vi "Get Request Type.vi"(8 "error in (no error)":errorcluster, 11 "SetProfileParameter in":refnum<class "SetProfileParameter.lvclass">) -> (0 "error out":errorcluster, 2 "Request Type":string, 3 "SetProfileParameter out":refnum<class "SetProfileParameter.lvclass">)   [LabVIEW 2022 SP3, in "obs-websocket-lv.lvlib" / "SetProfileParameter.lvclass"]
uses:
  SetProfileParameter.lvclass
  SetProfileParameter.lvclass/SetProfileParameter.ctl
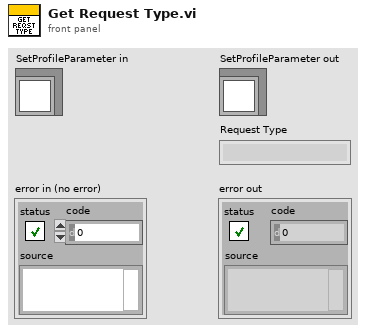
[diagram p1: front panel]
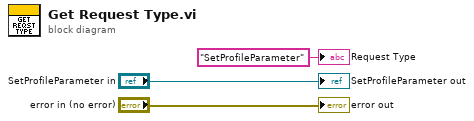
[diagram p0: block diagram]
diagram:
  "error out" <- "error in (no error)"
  "SetProfileParameter out" <- "SetProfileParameter in"
  "Request Type" <- "SetProfileParameter" ("Request Type")
